vi "TrimMsg.vi"(10 "Message":string) -> (2 "Msg":string)   [LabVIEW 2014]
panel:
  out "Ask User":bool
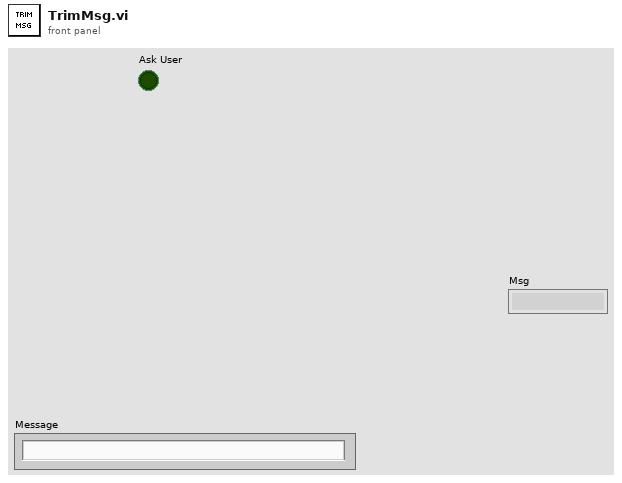
[diagram p1: front panel]
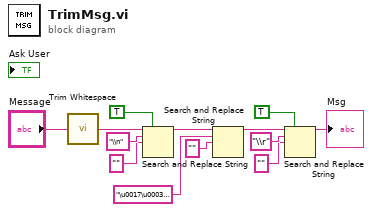
[diagram p0: block diagram]
diagram:
  n1 = call <vilib>:"Trim Whitespace.vi"("string"="Message") -> ("trimmed string"=w12:string)  [unwired: 1 in]
  n2 = Search and Replace String(replace all?=TRUE ("replace all? (F)"), input string=w12, search string="\\n" ("replace string (\"\")"), replace string="" ("replace string (\"\")")) -> (result string=w8:string)  [unwired: 4 in, 3 out]
  n3 = Search and Replace String(input string=w8, search string="\u0017\u0003\u0001", replace string="" ("replace string (\"\")")) -> (result string=w5:string)  [unwired: 5 in, 3 out]
  n4 = Search and Replace String(replace all?=TRUE ("replace all? (F)"), input string=w5, search string="\\r", replace string="" ("replace string (\"\")")) -> (result string=→"Msg":string)  [unwired: 4 in, 3 out]
